vi "Semaphore Strategy.vi"() -> ()   [LabVIEW 2010]
panel:
  out "Waveform Chart":dbl(graph)
  out "Profit":dbl format="%.6g"
  in  "Daily Balance":dbl
  in  "Daily Interest Gained":dbl
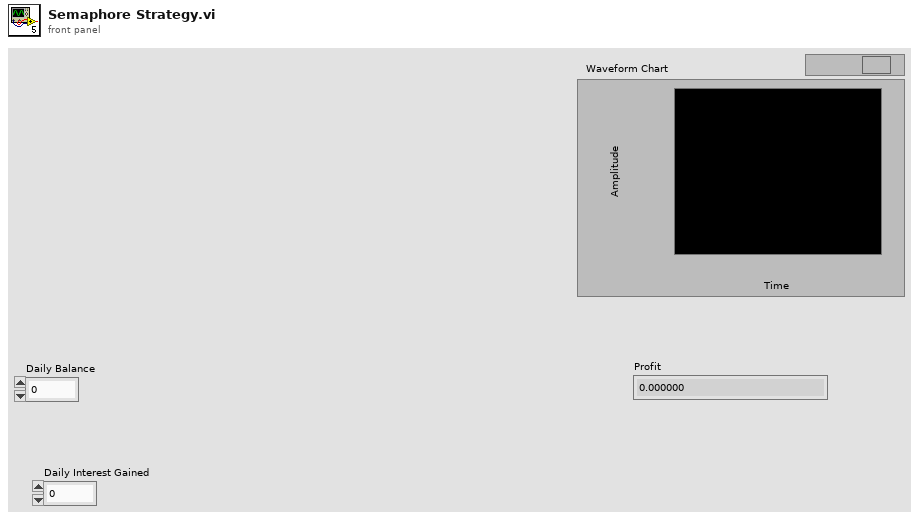
[diagram p1: front panel]
types:
  T1 = typedef "Semaphore RefNum" = refnum<k1>
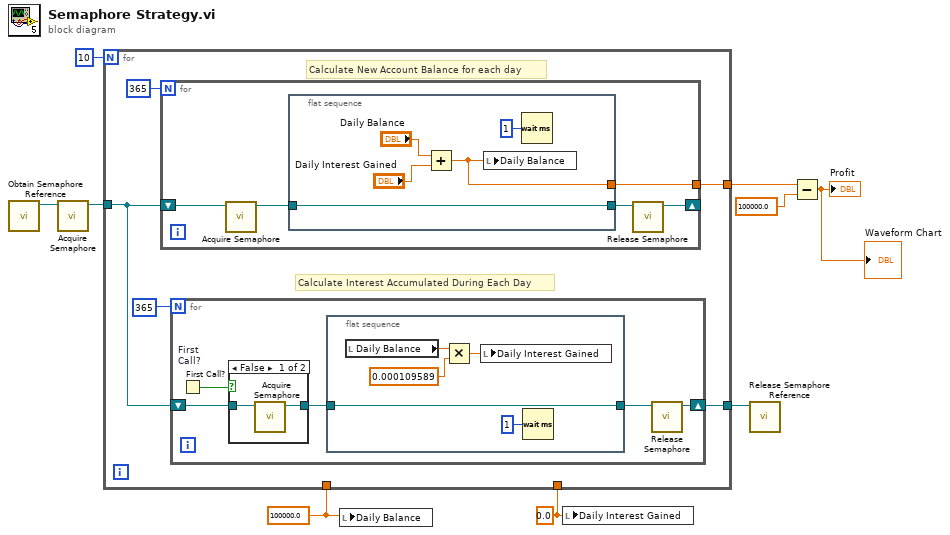
[diagram p0: block diagram]
diagram:
  w5 = 0.0 ("Daily Interest Gained")
  w6 = 100000.0 ("Daily Balance")
  n1 = call <vilib>:"Obtain Semaphore Reference.vi"() -> ("semaphore"=w3:T1)  [unwired: 5 in, 2 out]
  n2 = call <vilib>:"Acquire Semaphore.vi"("semaphore"=w3) -> ("semaphore out"=w2:T1)  [unwired: 4 in, 2 out]
  n3 = for {
    N: 10 -> [_]
    tunnel: [w13] -> w8
    tunnel: w6 -> [_]
    tunnel: w5 -> [_]
    tunnel: w2 -> [w12]
    tunnel: [w11] -> w4
    # "Calculate Interest Accumulated During Each Day"
    # "Calculate New Account Balance for each day"
    n4 = for {
      N: 365 -> [_]
      tunnel: [w32] -> w13
      shift-right: [w30] -> _
      shift-left: w12 -> [w31]
      n5 = call <vilib>:"Acquire Semaphore.vi"("semaphore"=w31) -> ("semaphore out"=w29:T1)  [unwired: 4 in, 2 out]
      n6 = flat-sequence {
        tunnel: [w37] -> w32
        tunnel: w29 -> [w33]
        tunnel: [w33] -> w28
        frame #0 {
          n7 = Add(x="Daily Balance", y="Daily Interest Gained") -> (x+y=w37:dbl)
          n8 = local write "Daily Balance"(w37) -> ()
          n9 = Wait (ms)(milliseconds to wait=u32 1) -> ()  [unwired: 1 out]
        }
      }
      n10 = call <vilib>:"Release Semaphore.vi"("semaphore"=w28) -> ("semaphore out"=w30:T1)  [unwired: 5 in, 1 out]
    }
    n11 = for {
      N: 365 -> [_]
      shift-right: [w18] -> w11
      shift-left: w12 -> [w19]
      n12 = First Call? "First\nCall?"() -> (First Call?: T/F=w17:bool)
      n13 = case shown="False" w17 {
        tunnel: w19 -> [w26 w27]
        tunnel: [w25 w27] -> w16
        frame False {
          n14 = call <vilib>:"Acquire Semaphore.vi"("semaphore"=w26) -> ("semaphore out"=w25:T1)  [unwired: 4 in, 2 out]
        }
        frame True {
        }
      }
      n15 = flat-sequence {
        tunnel: w16 -> [w21]
        tunnel: [w21] -> w15
        frame #0 {
          n16 = local read "Daily Balance"() -> (w24:dbl)
          n17 = Multiply(x=w24, y=0.000109589) -> (x*y=w22:dbl)
          n18 = local write "Daily Interest Gained"(w22) -> ()
          n19 = Wait (ms)(milliseconds to wait=u32 1) -> ()  [unwired: 1 out]
        }
      }
      n20 = call <vilib>:"Release Semaphore.vi"("semaphore"=w15) -> ("semaphore out"=w18:T1)  [unwired: 5 in, 1 out]
    }
  }
  n21 = local write "Daily Balance"(w6) -> ()
  n22 = local write "Daily Interest Gained"(w5) -> ()
  n23 = call <vilib>:"Release Semaphore Reference.vi"("semaphore"=w4) -> ()  [unwired: 9 in, 2 out]
  n24 = Subtract(x=w8, y=100000.0) -> (x-y=→"Profit" →"Waveform Chart":dbl)
